vi "Time Delay.vi"(8 "Error In":errorcluster, 10 "Delay(ms)":u32) -> (0 "Error Out":errorcluster)   [LabVIEW 2017]
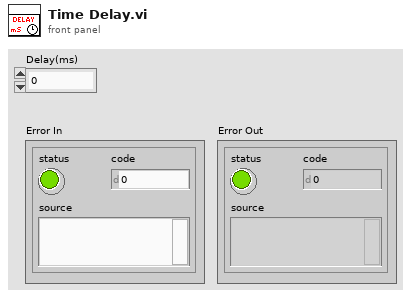
[diagram p1: front panel]
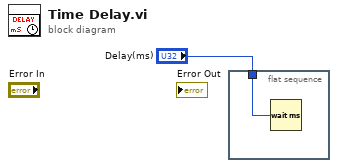
[diagram p0: block diagram]
diagram:
  n1 = flat-sequence {
    tunnel: "Delay(ms)" -> [w2]
    frame #0 {
      n2 = Wait (ms)(milliseconds to wait=w2) -> ()  [unwired: 1 out]
    }
  }
